vi "norm_mat.vi"(4 "vector":T1) -> (0 "magnitude":dbl, 1 "normalized vector":T1)   [LabVIEW 2013]
uses:
  <vilib>/Analysis/Matrix/Datatypes/RealMatrix.ctl
  <vilib>/Analysis/Matrix/Numeric/Multiply/Multiply - RM,R.vi
  <vilib>/Analysis/Matrix/NI_Matrix.lvlib
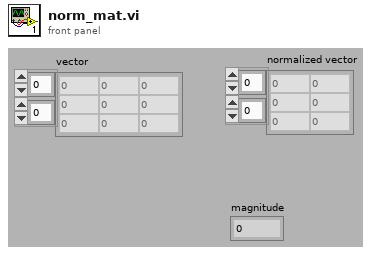
[diagram p1: front panel]
types:
  T1 = typedef "NI_Matrix.lvlib/RealMatrix.ctl" = dbl[][]
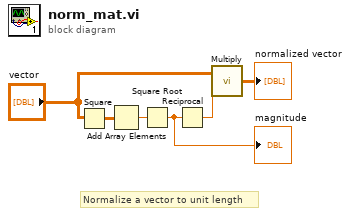
[diagram p0: block diagram]
diagram:
  # "Normalize a vector to unit length"
  n1 = Square(x="vector") -> (x^2=w6:T1)
  n2 = Add Array Elements(numeric array=w6) -> (sum=w5:dbl)
  n3 = Square Root(x=w5) -> (sqrt(x)=w1:dbl)
  "magnitude" <- w1
  n4 = Reciprocal(x=w1) -> (1/x=w4:dbl)
  n5 = call-poly <vilib>:"Multiply.vi"("Real Scalar c"=w4, "Real Matrix A"="vector") -> ("A * c"=→"normalized vector":T1)
